vi "HPS-17000 Custom Device.Async.vi"(10 "Parameters":variant, 11 "Process":refnum<class "Process.lvclass">) -> ()   [LabVIEW 2023, in "HPS-17000 Custom Device Engine.lvlib"]
uses:
  <vilib>/NI/NIVS Inline Async API/_VS Inline Async API/Process/Process.lvclass
  <vilib>/NI/NIVS Inline Async API/_VS Inline Async API/Process/Process.lvclass/Process.ctl
  <vilib>/NI/NIVS Inline Async API/_Data Access Engine/Access Type Classes/Read/Read.lvclass/Read.ctl
  <vilib>/NI/NIVS Inline Async API/_Data Access Engine/Access Type Classes/Write/Write.lvclass/Write.ctl
  <vilib>/NI/NIVS Inline Async API/_Data Access Engine/Data Access Engine/Methods/Read.Data.vi
  <vilib>/NI/NIVS Inline Async API/_Data Access Engine/Data Access Engine/Methods/Write.Data.vi
  <vilib>/NI/NIVS Inline Async API/_VS Inline Async API/Process/Data Member Access/Read Data Access.vi
  <vilib>/NI/NIVS Inline Async API/_VS Inline Async API/Error Handling Process/SubVIs/Error.ConvertArray.vi
  <vilib>/NI/NIVS Inline Async API/_Data Access Engine/Access Type Classes/Read/Read.ProcessData.vi
  <vilib>/NI/NIVS Inline Async API/_Data Access Engine/Access Type Classes/Write/Write.ProcessData.vi
  <vilib>/NI/NIVS Inline Async API/_Data Access Engine/Access Type Classes/Write/Write.Buffer.vi
  <vilib>/NI/NIVS Inline Async API/_Data Access Engine/Access Type Classes/Write/Write.Commit.vi
  <vilib>/NI/NIVS Inline Async API/_Data Access Engine/Data Access Engine/Methods/Write.Lookup.vi
  <vilib>/NI/NIVS Inline Async API/_Data Access Engine/Data Access Engine/Methods/Read.Lookup.vi
  <vilib>/NI/NIVS Inline Async API/_Data Access Engine/Data Access Engine/Data Access Engine.lvclass
  HPS-17000 Custom Device Engine.lvlib
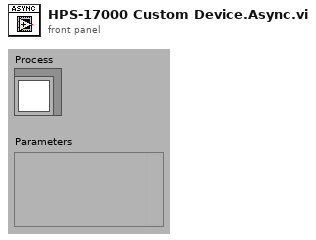
[diagram p1: front panel]
types:
  T1 = typedef "Data Access Engine.lvlib/Data Access Engine.lvclass/Write.DVR.ctl" = refnum<data-value>
  T2 = typedef "Data Access Engine.lvlib/Data Access Engine.lvclass/Read.DVR.ctl" = refnum<data-value>
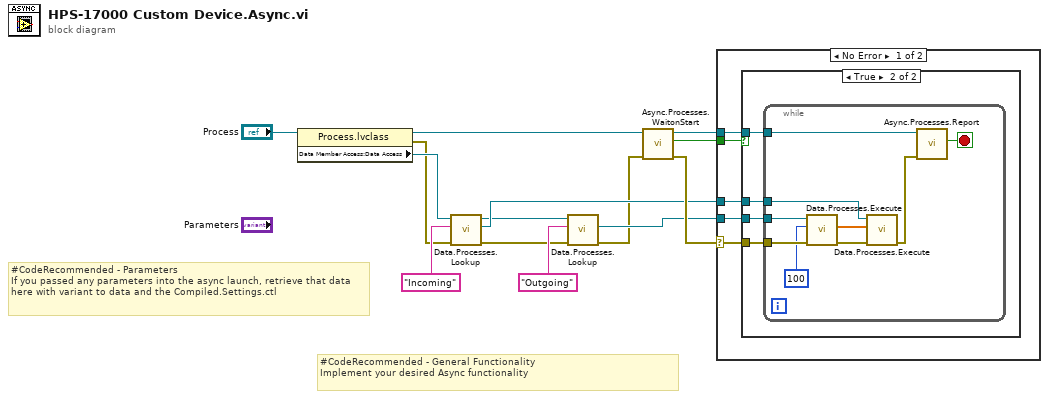
[diagram p0: block diagram]
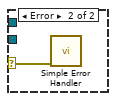
[diagram p3: hidden frame]
diagram:
  # "#CodeRecommended - General Functionality\nImplement your desired Async functionality"
  # "#CodeRecommended - Parameters\nIf you passed any parameters into the async launch, retrieve that data here with variant to data and the Compiled.Settings.ctl"
  n1 = property class="Process.lvclass"(reference="Process") -> (reference out=w3:refnum<class "Process.lvclass">, error out=w1:errorcluster, "Data Member Access:Data Access"=w2:refnum<class "Data Access Engine.lvclass">)  [unwired: 1 in]
  n2 = call-poly <vilib>:"Data.Processes.Lookup.vi"("error in (no error)"=w1, "Name"="Incoming", "Data Access API in"=w2) -> ("error out"=w8:errorcluster, "Ref"=w7:T1, "Data Access API out"=w6:refnum<class "Data Access Engine.lvclass">)  [unwired: 5 in, 1 out]
  n3 = call-poly <vilib>:"Data.Processes.Lookup.vi"("error in (no error)"=w8, "Name"="Outgoing", "Data Access API in"=w6) -> ("error out"=w5:errorcluster, "Ref"=w10:T2)  [unwired: 5 in, 2 out]
  n4 = call <vilib>:"Async.Processes.WaitonStart.vi"("error in (no error)"=w5, "Process"=w3) -> ("error out"=w12:errorcluster, "Execute"=w14:bool, "Process out"=w13:refnum<class "Process.lvclass">)  [unwired: 7 in]
  n5 = case shown="No Error" w12 {
    selector: w12 -> [w15 w33]
    tunnel: w14 -> [w19 _]
    tunnel: w13 -> [w18 _]
    tunnel: w7 -> [w17 _]
    tunnel: w10 -> [w16 _]
    frame No Error {
      n6 = case shown="True" w19 {
        tunnel: w15 -> [_ w20]
        tunnel: w18 -> [_ w21]
        tunnel: w16 -> [_ w23]
        tunnel: w17 -> [_ w22]
        frame False {
        }
        frame True {
          n7 = while {
            tunnel: w20 -> [w28]
            tunnel: w21 -> [w32]
            tunnel: w23 -> [w30]
            tunnel: w22 -> [w29]
            stop <- w31 stop-if-true
            n8 = call-poly <vilib>:"Data.Processes.Execute.vi"("error in (no error)"=w28, "timeout ms"=100, "Ref"=w30) -> ("error out"=w26:errorcluster, "Values"=w25:dbl[])  [unwired: 6 in, 1 out]
            n9 = call-poly <vilib>:"Data.Processes.Execute.vi"("error in (no error)"=w26, "Values"=w25, "Ref"=w29) -> ("error out"=w24:errorcluster)  [unwired: 8 in]
            n10 = call <vilib>:"Async.Processes.Report.vi"("Error"=w24, "Process in"=w32) -> ("Stop"=w31:bool)  [unwired: 8 in, 1 out]
          }
        }
      }
    }
    frame Error {
      n11 = call <vilib>:"Simple Error Handler.vi"("error in (no error)"=w33) -> ()  [unwired: 4 in, 5 out]
    }
  }
